vi "Generic command handler.vi"(8 "error in (no error)":errorcluster, 10 "Message in":refnum<class "GenericMessage.lvclass">, 11 "ConfocalStage in":refnum<class "ConfocalStage.lvclass">) -> (0 "error out":errorcluster, 2 "value":string, 3 "ConfocalStage out":refnum<class "ConfocalStage.lvclass">)   [LabVIEW 2012, in "ConfocalStage.lvclass"]
doc: "The generic_command_handler processes the command 'generic'. Commands which are not part of the predefined list of commands fall under the 'generic' command for special activity."
uses:
  ConfocalStage.lvclass
  <vilib>/Distrio/Murmex/GenericMessage/GenericMessage.lvclass
  <vilib>/Distrio/Murmex/Murmex/Murmex.lvclass
  ConfocalStage.lvclass/ConfocalStage.ctl
  <vilib>/Distrio/Murmex/ProceedMessage/ProceedMessage.lvclass
  <vilib>/Distrio/Murmex/Message/Message.lvclass
panel:
  # "This method is called when the GENERIC\ntrigger is sent. \n\nOverride this method when your component needs to\nrespond to this trigger. \n\nCall parent for proper implementation"
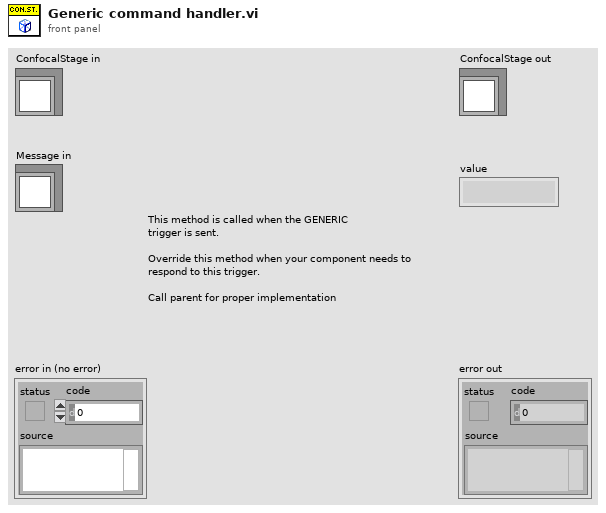
[diagram p1: front panel]
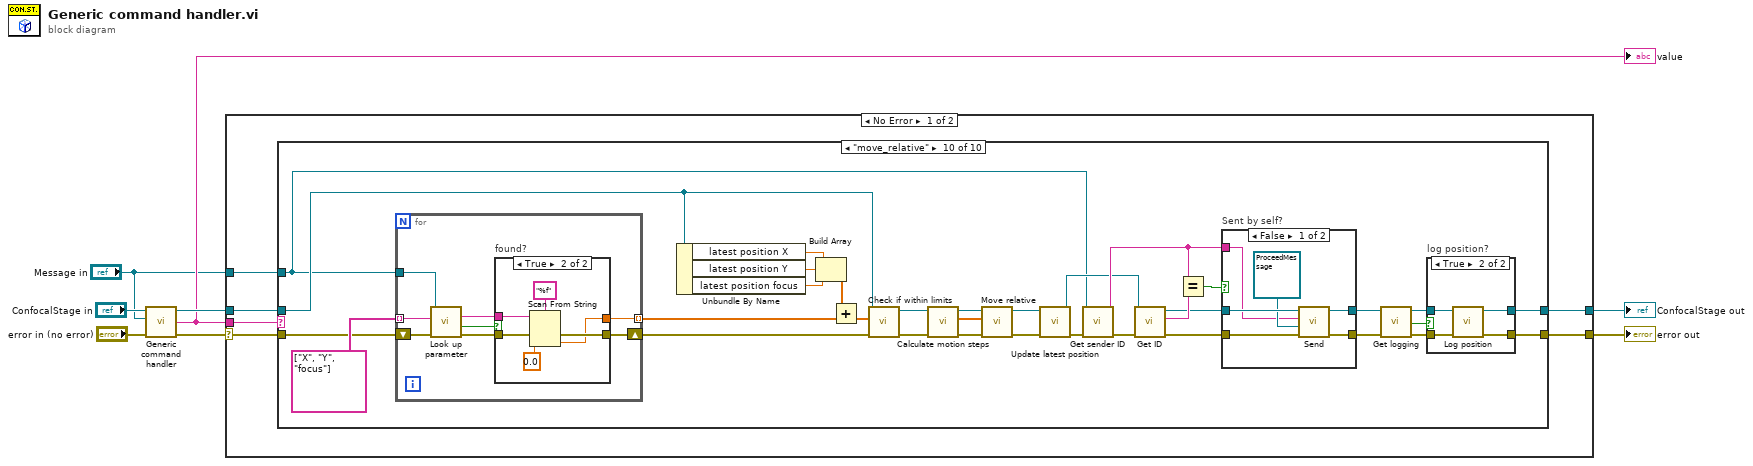
[diagram p0: block diagram]
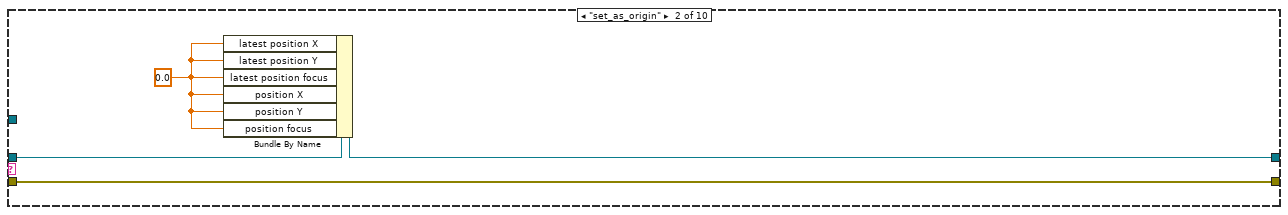
[diagram p3: hidden frame]
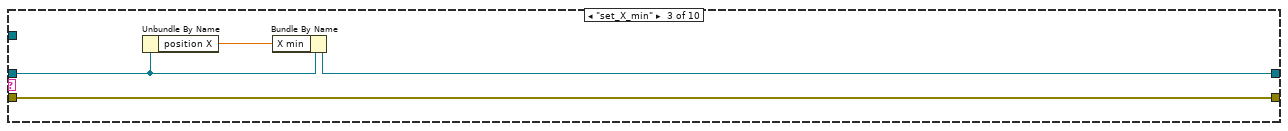
[diagram p4: hidden frame]
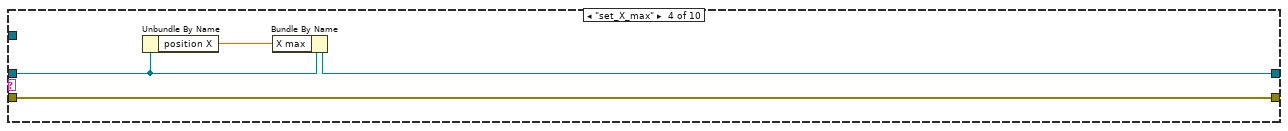
[diagram p5: hidden frame]
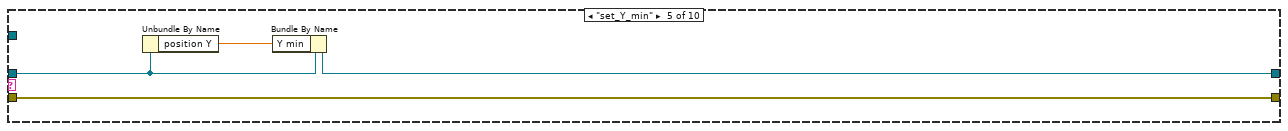
[diagram p6: hidden frame]
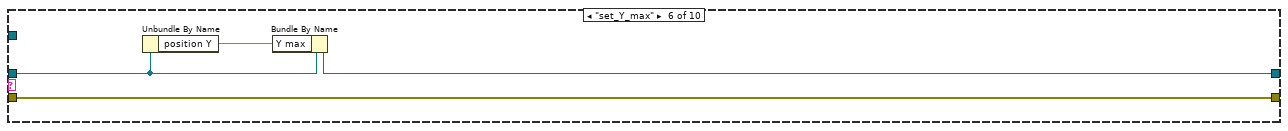
[diagram p7: hidden frame]
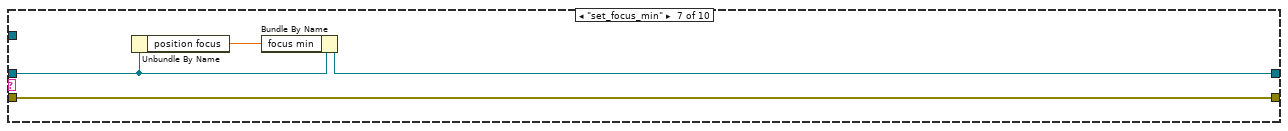
[diagram p8: hidden frame]
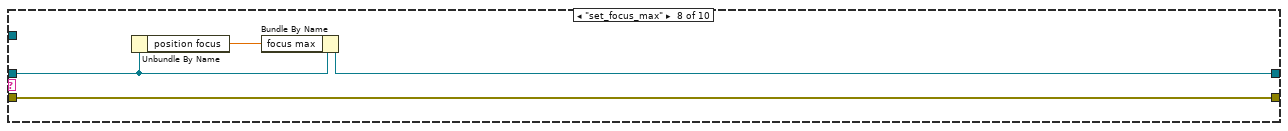
[diagram p9: hidden frame]
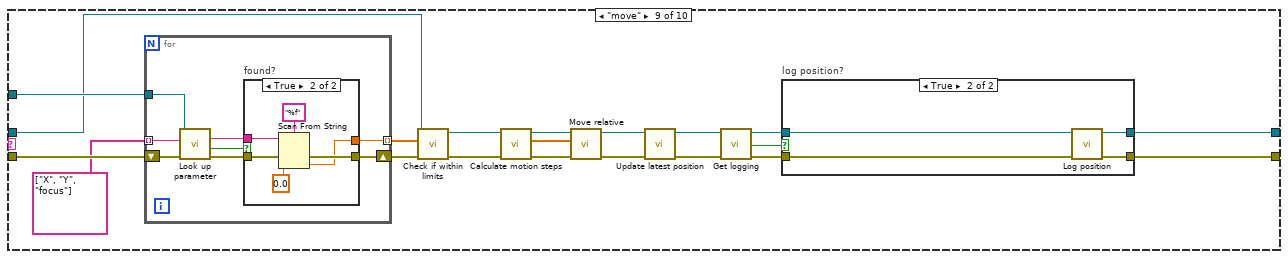
[diagram p10: hidden frame]
diagram:
  n1 = call-parent "Generic command handler.vi"("error in (no error)"="error in (no error)", "Message in"="Message in", "Murmex in"="ConfocalStage in") -> ("error out"=w6:errorcluster, "value"=w2:string, "Murmex out"=w5:refnum<class "ConfocalStage.lvclass">)  [unwired: 6 in]
  "value" <- w2
  n2 = case shown="No Error" w6 {
    selector: w6 -> [w12 w148]
    tunnel: w5 -> [w10 w149]
    tunnel: [w11 w149] -> w4
    tunnel: [w13 w148] -> w3
    tunnel: w2 -> [w14 _]
    tunnel: "Message in" -> [w9 _]
    frame No Error {
      n3 = case shown="\"move_relative\"" w14 {
        tunnel: [w16 w18 w21 w25 w29 w33 w37 w41 w45 w99] -> w13
        tunnel: w12 -> [w16 w18 w21 w25 w29 w33 w37 w41 w64 w109]
        tunnel: [w15 w19 w23 w27 w31 w35 w39 w43 w46 w97] -> w11
        tunnel: w10 -> [w15 w20 w24 w28 w32 w36 w40 w44 w59 w108]
        tunnel: w9 -> [_ _ _ _ _ _ _ _ w63 w86]
        frame Default {
        }
        frame "set_as_origin" {
          w17 = 0.0 ("runtime.position X")
          n4 = Bundle By Name(cluster=w20, "latest position X"=w17, "latest position Y"=w17, "latest position focus"=w17, "position X"=w17, "position Y"=w17, "position focus"=w17) -> (w19:refnum<class "ConfocalStage.lvclass">)
        }
        frame "set_X_min" {
          n5 = Unbundle By Name(w24) -> ("position X"=w22:dbl)
          n6 = Bundle By Name(cluster=w24, "X min"=w22) -> (w23:refnum<class "ConfocalStage.lvclass">)
        }
        frame "set_X_max" {
          n7 = Unbundle By Name(w28) -> ("position X"=w26:dbl)
          n8 = Bundle By Name(cluster=w28, "X max"=w26) -> (w27:refnum<class "ConfocalStage.lvclass">)
        }
        frame "set_Y_min" {
          n9 = Unbundle By Name(w32) -> ("position Y"=w30:dbl)
          n10 = Bundle By Name(cluster=w32, "Y min"=w30) -> (w31:refnum<class "ConfocalStage.lvclass">)
        }
        frame "set_Y_max" {
          n11 = Unbundle By Name(w36) -> ("position Y"=w34:dbl)
          n12 = Bundle By Name(cluster=w36, "Y max"=w34) -> (w35:refnum<class "ConfocalStage.lvclass">)
        }
        frame "set_focus_min" {
          n13 = Unbundle By Name(w40) -> ("position focus"=w38:dbl)
          n14 = Bundle By Name(cluster=w40, "focus min"=w38) -> (w39:refnum<class "ConfocalStage.lvclass">)
        }
        frame "set_focus_max" {
          n15 = Unbundle By Name(w44) -> ("position focus"=w42:dbl)
          n16 = Bundle By Name(cluster=w44, "focus max"=w42) -> (w43:refnum<class "ConfocalStage.lvclass">)
        }
        frame "move" {
          n17 = for {
            tunnel: w63 -> [w74]
            shift-right: [w73] -> w61
            shift-left: w64 -> [w75]
            tunnel: string[] ["X", "Y", "focus"] -> [w72] mode=indexing
            tunnel: [w71] -> w60 mode=indexing
            n18 = call <vilib>:"Look up parameter.vi"("error in (no error)"=w75, "name"=w72, "Message in"=w74) -> ("error out"=w77:errorcluster, "found?"=w78:bool, "key"=w76:string)  [unwired: 5 in, 1 out]
            n19 = case "found?" shown="True" w78 {
              tunnel: w77 -> [w79 w84]
              tunnel: w76 -> [_ w83]
              tunnel: [w79 w81] -> w73
              tunnel: [_ w80] -> w71
              frame False {
              }
              frame True {
                n20 = Scan From String(format string="%f", input string=w83, error in=w84, default 1=0.0 ("default value 1")) -> (error out=w81:errorcluster, output 1=w80:dbl)  [unwired: 1 in, 2 out]
              }
            }
          }
          n21 = call-dynamic "Check if within limits.vi"("error in (no error)"=w61, "Target position array"=w60, "ConfocalStage in"=w59) -> ("error out"=w57:errorcluster, "ConfocalStage out"=w58:refnum<class "ConfocalStage.lvclass">)  [unwired: 6 in, 1 out]
          n22 = call-dynamic "Calculate motion steps.vi"("error in (no error)"=w57, "ConfocalStage in"=w58) -> ("error out"=w54:errorcluster, "Relative motion array"=w55:dbl[], "ConfocalStage out"=w56:refnum<class "ConfocalStage.lvclass">)  [unwired: 7 in]
          n23 = call-dynamic "Move relative.vi"("error in (no error)"=w54, "Move array"=w55, "ConfocalStage in"=w56) -> ("error out"=w53:errorcluster, "ConfocalStage out"=w52:refnum<class "ConfocalStage.lvclass">)  [unwired: 7 in]
          n24 = call-dynamic "Update latest position.vi"("error in (no error)"=w53, "ConfocalStage in"=w52) -> ("error out"=w47:errorcluster, "ConfocalStage out"=w48:refnum<class "ConfocalStage.lvclass">)  [unwired: 8 in]
          n25 = call-dynamic "Get logging.vi"("error in (no error)"=w47, "ConfocalStage in"=w48) -> ("error out"=w50:errorcluster, "logging?"=w51:bool, "ConfocalStage out"=w49:refnum<class "ConfocalStage.lvclass">)  [unwired: 7 in]
          n26 = case "log position?" shown="True" w51 {
            tunnel: w50 -> [w66 w70]
            tunnel: [w66 w67] -> w45
            tunnel: [w65 w68] -> w46
            tunnel: w49 -> [w65 w69]
            frame False {
            }
            frame True {
              n27 = call-dynamic "Log position.vi"("error in (no error)"=w70, "ConfocalStage in"=w69) -> ("error out"=w67:errorcluster, "ConfocalStage out"=w68:refnum<class "ConfocalStage.lvclass">)  [unwired: 8 in]
            }
          }
        }
        frame "move_relative" {
          n28 = for {
            tunnel: w86 -> [w136]
            shift-right: [w135] -> w117
            shift-left: w109 -> [w137]
            tunnel: string[] ["X", "Y", "focus"] -> [w134] mode=indexing
            tunnel: [w133] -> w104 mode=indexing
            n29 = call <vilib>:"Look up parameter.vi"("error in (no error)"=w137, "name"=w134, "Message in"=w136) -> ("error out"=w139:errorcluster, "found?"=w140:bool, "key"=w138:string)  [unwired: 5 in, 1 out]
            n30 = case "found?" shown="True" w140 {
              tunnel: w139 -> [w141 w146]
              tunnel: w138 -> [_ w145]
              tunnel: [w141 w143] -> w135
              tunnel: [_ w142] -> w133
              frame False {
              }
              frame True {
                n31 = Scan From String(format string="%f", input string=w145, error in=w146, default 1=0.0 ("default value 1")) -> (error out=w143:errorcluster, output 1=w142:dbl)  [unwired: 1 in, 2 out]
              }
            }
          }
          n32 = Unbundle By Name(w108) -> ("latest position X"=w106:dbl, "latest position Y"=w107:dbl, "latest position focus"=w105:dbl)
          n33 = Build Array(w106, w107, w105) -> (w103:dbl[])
          n34 = Add(x=w103, y=w104) -> (x+y=w102:dbl[])
          n35 = call-dynamic "Check if within limits.vi"("error in (no error)"=w117, "Target position array"=w102, "ConfocalStage in"=w108) -> ("error out"=w115:errorcluster, "ConfocalStage out"=w116:refnum<class "ConfocalStage.lvclass">)  [unwired: 6 in, 1 out]
          n36 = call-dynamic "Calculate motion steps.vi"("error in (no error)"=w115, "ConfocalStage in"=w116) -> ("error out"=w112:errorcluster, "Relative motion array"=w113:dbl[], "ConfocalStage out"=w114:refnum<class "ConfocalStage.lvclass">)  [unwired: 7 in]
          n37 = call-dynamic "Move relative.vi"("error in (no error)"=w112, "Move array"=w113, "ConfocalStage in"=w114) -> ("error out"=w111:errorcluster, "ConfocalStage out"=w110:refnum<class "ConfocalStage.lvclass">)  [unwired: 7 in]
          n38 = call-dynamic "Update latest position.vi"("error in (no error)"=w111, "ConfocalStage in"=w110) -> ("error out"=w90:errorcluster, "ConfocalStage out"=w89:refnum<class "ConfocalStage.lvclass">)  [unwired: 8 in]
          n39 = call <vilib>:"Get sender ID.vi"("error in (no error)"=w90, "Message in"=w86) -> ("error out"=w96:errorcluster, "sender"=w91:string)  [unwired: 7 in, 1 out]
          n40 = call <vilib>:"Get ID.vi"("error in (no error)"=w96, "Murmex in"=w89) -> ("error out"=w93:errorcluster, "component id"=w95:string, "Murmex out"=w92:refnum<class "ConfocalStage.lvclass">)  [unwired: 7 in]
          n41 = Equal?(x=w91, y=w95) -> (x = y?=w94:bool)
          n42 = case "Sent by self?" shown="False" w94 {
            tunnel: [w121 w126] -> w88
            tunnel: w93 -> [w124 w126]
            tunnel: [w122 w125] -> w87
            tunnel: w92 -> [w123 w125]
            tunnel: w91 -> [w119 _]
            frame False {
              n43 = call <vilib>:"Send.vi"("error in (no error)"=w124, "Message"=refnum<class "ProceedMessage.lvclass"> refnum ("ProceedMessage"), "recipient"=w119, "Murmex in"=w123) -> ("error out"=w121:errorcluster, "Murmex out"=w122:refnum<class "ConfocalStage.lvclass">)  [unwired: 6 in]
            }
            frame True {
            }
          }
          n44 = call-dynamic "Get logging.vi"("error in (no error)"=w88, "ConfocalStage in"=w87) -> ("error out"=w100:errorcluster, "logging?"=w101:bool, "ConfocalStage out"=w98:refnum<class "ConfocalStage.lvclass">)  [unwired: 7 in]
          n45 = case "log position?" shown="True" w101 {
            tunnel: w100 -> [w128 w132]
            tunnel: [w128 w129] -> w99
            tunnel: [w127 w130] -> w97
            tunnel: w98 -> [w127 w131]
            frame False {
            }
            frame True {
              n46 = call-dynamic "Log position.vi"("error in (no error)"=w132, "ConfocalStage in"=w131) -> ("error out"=w129:errorcluster, "ConfocalStage out"=w130:refnum<class "ConfocalStage.lvclass">)  [unwired: 8 in]
            }
          }
        }
      }
    }
    frame Error {
    }
  }
  "error out" <- w3
  "ConfocalStage out" <- w4
